vi "Register Entity.vi"(8 "error in (no error)":errorcluster, 10 "Entity":refnum<class "Entity.lvclass">, 11 "Entity Manager in":refnum<class "Entity Manager.lvclass">) -> (0 "error out":errorcluster, 2 "Table Name":string, 3 "Entity Manager out":refnum<class "Entity Manager.lvclass">)   [LabVIEW 2022 SP3, in "Conditum.lvlib" / "Entity Manager.lvclass"]
uses:
  Entity Manager.lvclass
  Entity Manager.lvclass/Entity Manager.ctl
  Entity/Entity.lvclass
  Database Platform/Database Platform.lvclass
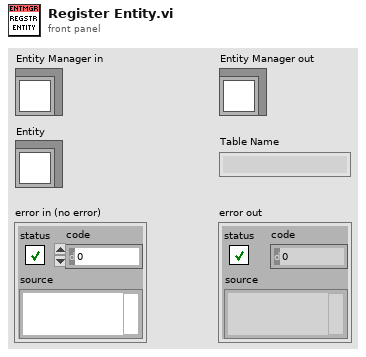
[diagram p1: front panel]
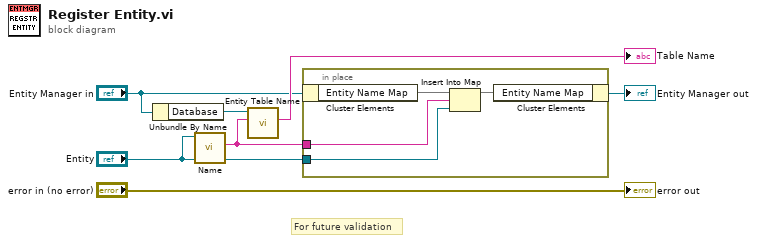
[diagram p0: block diagram]
diagram:
  # "For future validation"
  n1 = Unbundle By Name("Entity Manager in") -> ("Database"=w2:refnum<class "Database Platform.lvclass">)
  n2 = call-dynamic "Name.vi"("Entity in"="Entity") -> ("Name"=w1:string)  [unwired: 10 in]
  n3 = call-dynamic "Entity Table Name.vi"("Entity Name"=w1, "Database in"=w2) -> ("Table Name"=→"Table Name":string)  [unwired: 9 in]
  n4 = in-place {
    in-place-border: "Entity" -> [w10]
    in-place-border: w1 -> [w8]
    n5 = in-place-cluster #1("Entity Manager in") -> ("Entity Name Map"=w11:map{string, refnum<class "Entity.lvclass">})
    n6 = Insert Into Map(map in=w11, key=w8, value=w10) -> (map out=w9:map{string, refnum<class "Entity.lvclass">})  [unwired: 2 out]
    n7 = in-place-cluster #1("Entity Name Map"=w9) -> (→"Entity Manager out":refnum<class "Entity Manager.lvclass">)
  }
  "error out" <- "error in (no error)"
